vi "Receive.vi"(8 "error in":errorcluster, 11 "HSU MCU V2 Monitor CFG in":refnum<class "HSU MCU V2 Monitor CFG.lvclass">) -> (0 "error out":errorcluster, 3 "HSU MCU V2 Monitor CFG out":refnum<class "HSU MCU V2 Monitor CFG.lvclass">)   [LabVIEW 2023]
uses:
  Protocols/ICommunicate/ICAN.lvclass
  HSU MCU V2 Monitor CFG.lvclass
  D:/git/HAL/HAL GOOP4/Configuration/Configuration JSON/Configuration JSON Base/CFG JSON.lvclass
  D:/git/HAL/HAL GOOP4/Interfaces/IConfigure/IConfigure.lvclass
  D:/git/HAL/HAL GOOP4/Devices/HSU MCU V2 Monitor CFG/HSU MCU V2 Monitor CFG.lvclass
  <instrlib>/KDI Digital Instrumentation/API_for_PCAN_BASIC_FD/CAN MSG Cluster.ctl
panel:
  in  "CAN_Message out":T1={"ID"=0, "MSG type"=0, "DLC"=0, "DATA"=[0, 0, 0, 0, 0, 0, 0, 0]} {"MSG type" format="%x"; "ID" format="%.0x"}
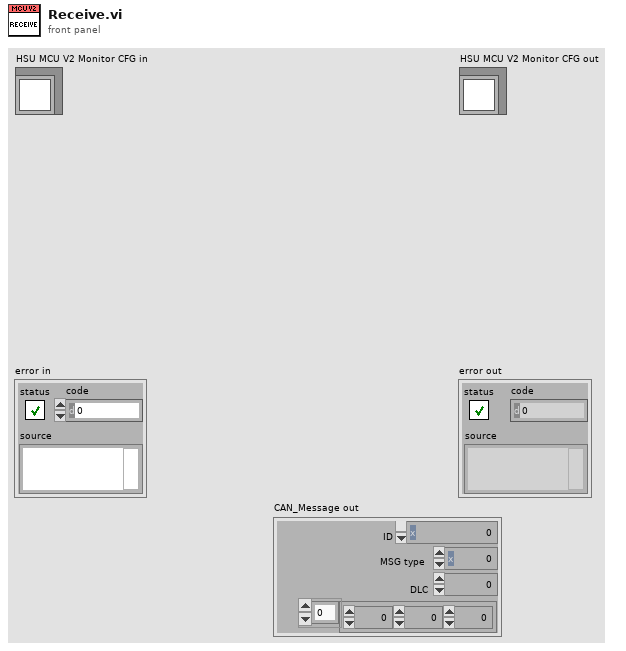
[diagram p1: front panel]
types:
  T1 = typedef "CAN MSG Cluster.ctl" = cluster{"ID":u32, "MSG type":u8, "DLC":u8, "DATA":u8[]}
  T2 = typedef "TPCANTimestamp.ctl" = cluster{"millis overflow":u16, "millis ":u32, "micros":u16}
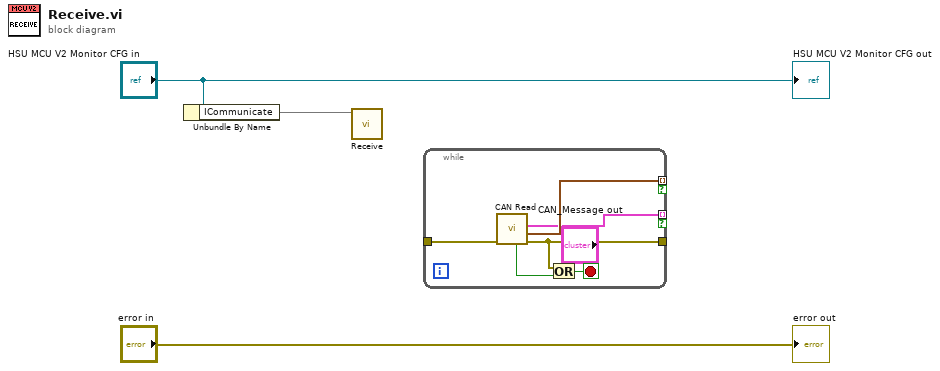
[diagram p0: block diagram]
diagram:
  n1 = Unbundle By Name("HSU MCU V2 Monitor CFG in") -> ("ICommunicate"=w2)
  n2 = call-dynamic "Receive.vi"("ICommunicate in"=w2) -> ()  [unwired: 8 in, 3 out]
  n3 = while {
    tunnel: _ -> [w10]
    tunnel: [w7] -> _
    tunnel: [w6] -> _ mode=indexing if=_
    tunnel: [w5] -> w1 mode=indexing if=_
    stop <- w9 stop-if-true
    n4 = call <instrlib>:"CAN Read.vi"("error in (no error)"=w10) -> ("error out"=w7:errorcluster, "TPCANTimestamp out"=w6:T2, "CAN_Message out"=w5:T1, "rcv queue empty"=w8:bool)  [unwired: 6 in, 1 out]
    n5 = Or(x=w7, y=w8) -> (x .or. y?=w9:bool)
  }
  "error out" <- "error in"
  "HSU MCU V2 Monitor CFG out" <- "HSU MCU V2 Monitor CFG in"
